vi "Ring-Set nicely by string.vi"(0 "Ring in":refnum<vi>, 5 "error in (no error)":errorcluster, 7 "Device":string, 9 "Default (0)":i32, 11 "Strings []":string[](array[string])) -> (4 "reference out":refnum<vi>, 6 "error out":errorcluster, 8 "Index":i32, 10 "Selection":string, 14 "next":i32)   [LabVIEW 2020]
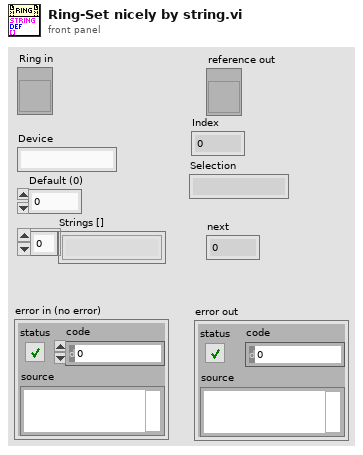
[diagram p1: front panel]
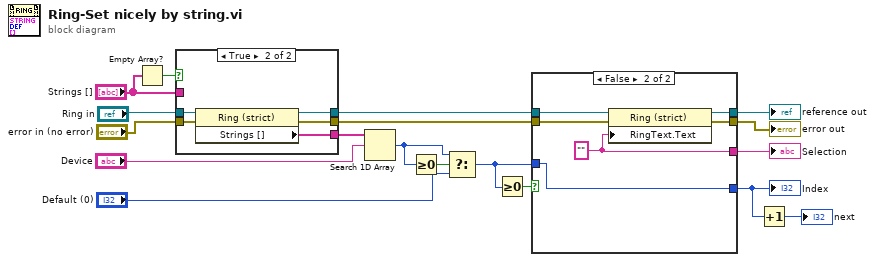
[diagram p0: block diagram]
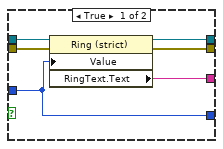
[diagram p2: hidden frame]
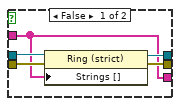
[diagram p3: hidden frame]
diagram:
  n1 = Empty Array?(array="Strings []") -> (empty?=w8:bool)
  n2 = case shown="True" w8 {
    tunnel: [w19 w28] -> w17
    tunnel: "Ring in" -> [w21 w27]
    tunnel: [w22 w26] -> w15
    tunnel: "error in (no error)" -> [w20 w25]
    tunnel: [w23 w24] -> w11
    tunnel: "Strings []" -> [w19 _]
    frame False {
      n3 = property class="Ring (strict)"(reference=w21, error in=w20, "Strings []"=w19) -> (reference out=w22:refnum<vi>, error out=w23:errorcluster)
    }
    frame True {
      n4 = property class="Ring (strict)"(reference=w27, error in=w25) -> (reference out=w26:refnum<vi>, error out=w24:errorcluster, "Strings []"=w28:string[])
    }
  }
  n5 = Search 1D Array(1D array=w17, element="Device") -> (index of element=w13:i32)  [unwired: 1 in]
  n6 = Greater Or Equal To 0?(x=w13) -> (x >= 0?=w14:bool)
  n7 = Select(t=w13, s=w14, f="Default (0)") -> (s? t:f=w3:i32)
  n8 = Greater Or Equal To 0?(x=w3) -> (x >= 0?=w4:bool)
  n9 = case shown="False" w4 {
    tunnel: w15 -> [w34 w40]
    tunnel: w3 -> [w29 w36]
    tunnel: w11 -> [w33 w39]
    tunnel: [w32 w38] -> w10
    tunnel: [w31 w37] -> w9
    tunnel: [w30 w35] -> w6
    tunnel: [w29 w36] -> w2
    frame True {
      n10 = property class="Ring (strict)"(reference=w34, error in=w33, "Value"=w29) -> (reference out=w31:refnum<vi>, error out=w32:errorcluster, "RingText.Text"=w30:string)
    }
    frame False {
      w35 = ""
      n11 = property class="Ring (strict)"(reference=w40, error in=w39, "RingText.Text"=w35) -> (reference out=w37:refnum<vi>, error out=w38:errorcluster)
    }
  }
  "error out" <- w10
  "reference out" <- w9
  "Index" <- w2
  "Selection" <- w6
  n12 = Increment(x=w2) -> (x+1=→"next":i32)
